vi "mark_10_config_panel.vi"(8 "Error In":errorcluster, 11 "Mark-10 Settings":T1) -> (0 "Error Out":errorcluster, 3 "Mark-10 Settings 2":T1)   [LabVIEW 2017]
uses:
  mark_10_setting_1.ctl
panel:
  in  "Cancel Button":bool
  in  "OK Button":bool
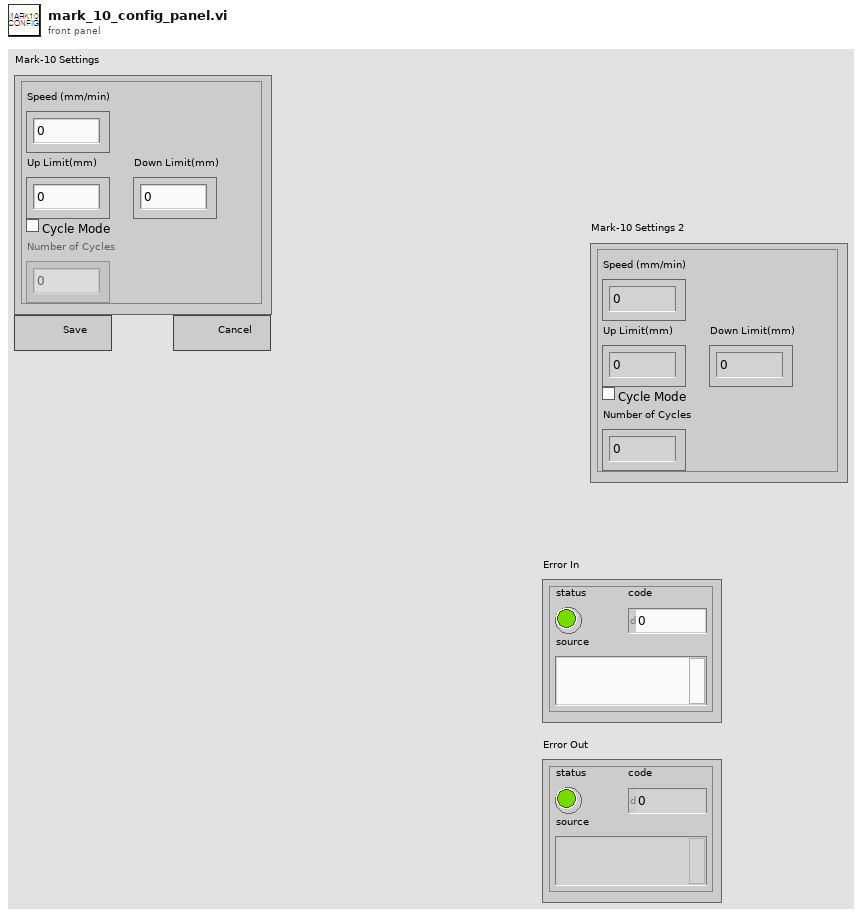
[diagram p1: front panel]
types:
  T1 = typedef "mark_10_setting_1.ctl" = cluster{"Speed (mm/min)":dbl, "Up Limit(mm)":dbl, "Down Limit(mm)":dbl, "Cycle Mode":bool, "Number of Cycles":i32, "IsConfigured":bool}
  T2 = enum8{"Enabled", "Disabled", "Disabled and Grayed Out"}
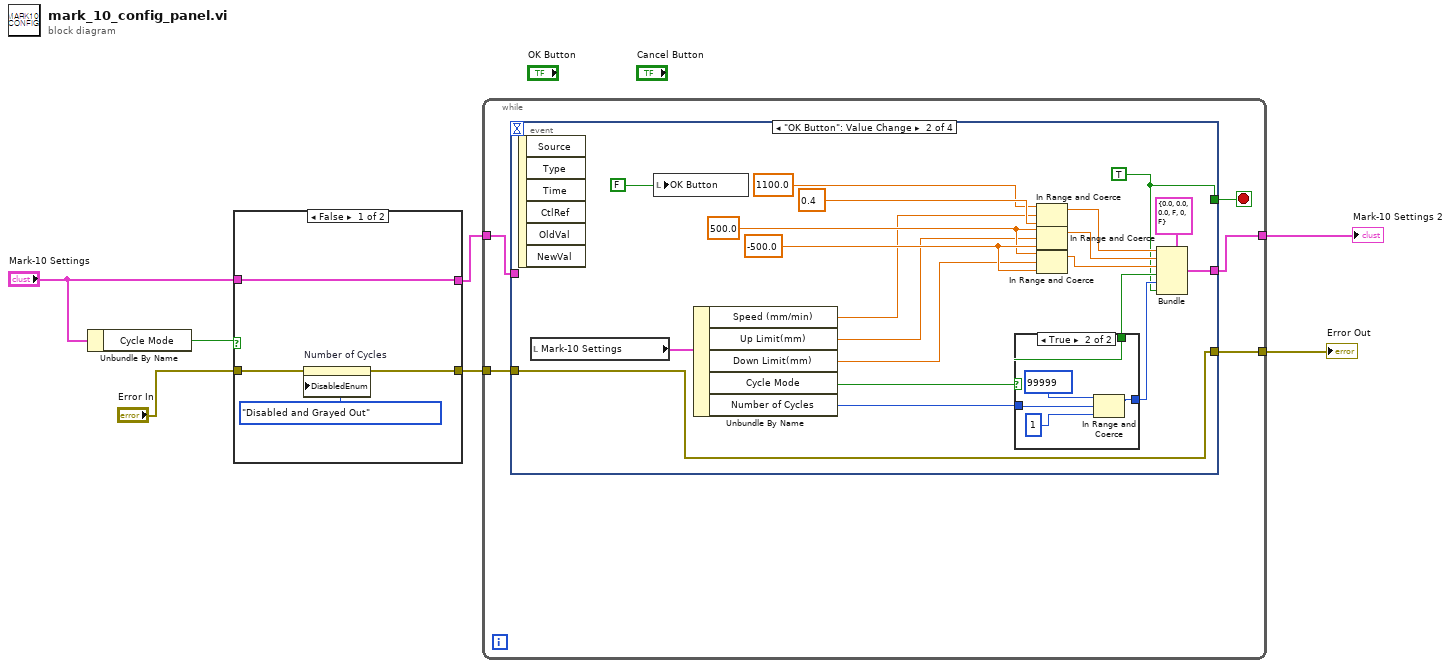
[diagram p0: block diagram]
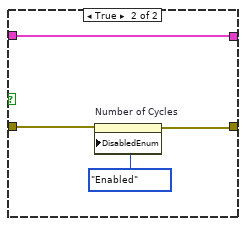
[diagram p2: hidden frame]
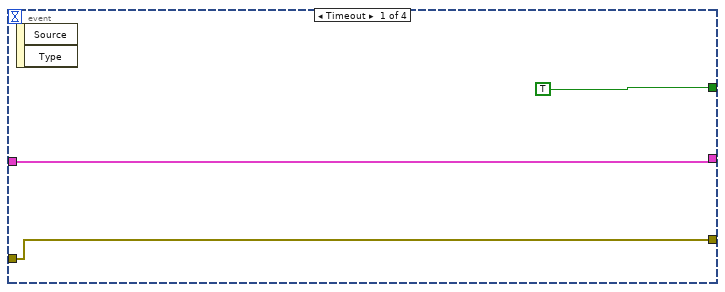
[diagram p3: hidden frame]
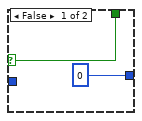
[diagram p4: hidden frame]
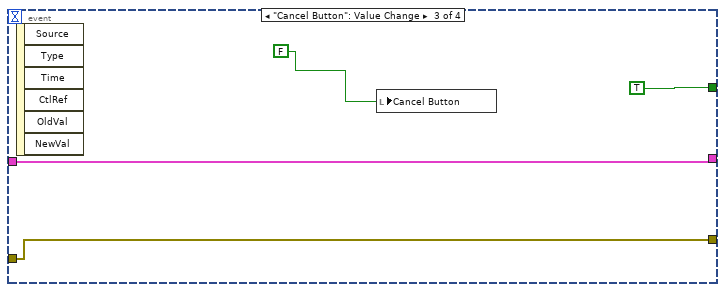
[diagram p5: hidden frame]
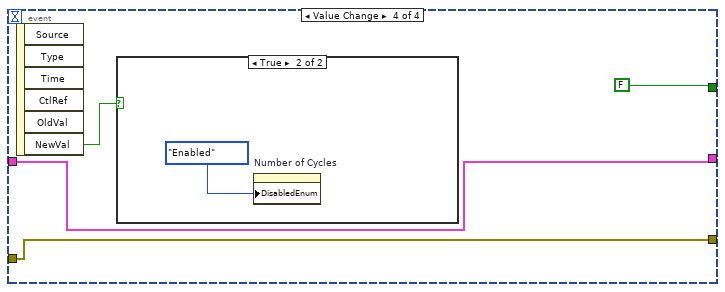
[diagram p6: hidden frame]
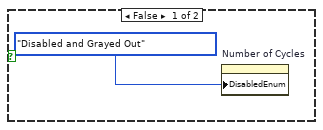
[diagram p7: hidden frame]
diagram:
  n1 = Unbundle By Name("Mark-10 Settings") -> ("Cycle Mode"=w6:bool)
  n2 = case shown="False" w6 {
    tunnel: [w10 w14] -> w4
    tunnel: "Mark-10 Settings" -> [w10 w14]
    tunnel: "Error In" -> [w9 w13]
    tunnel: [w8 w12] -> w2
    frame False {
      n3 = property on="Number of Cycles" class="DigNum (strict)"(error in=w9, "DisabledEnum"=T2."Disabled and Grayed Out" ("Disabled")) -> (error out=w8:errorcluster)  [unwired: 1 in, 1 out]
    }
    frame True {
      n4 = property on="Number of Cycles" class="DigNum (strict)"(error in=w13, "DisabledEnum"=T2."Enabled" ("Disabled")) -> (error out=w12:errorcluster)  [unwired: 1 in, 1 out]
    }
  }
  n5 = while {
    tunnel: w4 -> [w18]
    tunnel: [w20] -> w7
    tunnel: w2 -> [w17]
    tunnel: [w16] -> w1
    stop <- w19 stop-if-true
    n6 = event shown="[1] \"OK Button\": Value Change" {
      selector: _ -> [_ _ _ _]
      dyn-events: _ -> [_ _ _ _]
      timeout: _ -> [_ _ _ _]
      tunnel: [TRUE w24 TRUE FALSE] -> w19
      tunnel: [w22 w38 w52 w56] -> w20
      tunnel: w18 -> [w22 _ w52 w56]
      tunnel: w17 -> [w21 w36 w51 w55]
      tunnel: [w21 w36 w51 w55] -> w16
      event Timeout {
        n7 = event-data() -> ()  [unwired: 1 in, 2 out]
      }
      event "OK Button": Value Change {
        w42 = -500.0
        w41 = 500.0
        w24 = TRUE
        n8 = event-data() -> ()  [unwired: 1 in, 6 out]
        n9 = local read "Mark-10 Settings"() -> (w35:T1)
        n10 = local write "OK Button"(FALSE) -> ()
        n11 = Unbundle By Name(w35) -> ("Speed (mm/min)"=w30:dbl, "Up Limit(mm)"=w31:dbl, "Down Limit(mm)"=w32:dbl, "Cycle Mode"=w33:bool, "Number of Cycles"=w34:i32)
        n12 = case shown="True" w33 {
          selector: w33 -> [w44 w46]
          tunnel: [0 w50] -> w29
          tunnel: w34 -> [_ w47]
          tunnel: [w44 w46] -> w28
          frame False {
          }
          frame True {
            n13 = In Range and Coerce(upper limit=99999, x=w47, lower limit=1) -> (coerced(x)=w50:i32)  [unwired: 1 out]
          }
        }
        n14 = In Range and Coerce(upper limit=1100.0, x=w30, lower limit=0.4) -> (coerced(x)=w27:dbl)  [unwired: 1 out]
        n15 = In Range and Coerce(upper limit=w41, x=w31, lower limit=w42) -> (coerced(x)=w26:dbl)  [unwired: 1 out]
        n16 = In Range and Coerce(upper limit=w41, x=w32, lower limit=w42) -> (coerced(x)=w25:dbl)  [unwired: 1 out]
        n17 = Bundle(cluster=T1 {"Speed (mm/min)"=0.0, "Up Limit(mm)"=0.0, "Down Limit(mm)"=0.0, "Cycle Mode"=FALSE, "Number of Cycles"=0, "IsConfigured"=FALSE} ("Mark-10 Settings"), "Speed (mm/min)"=w27, "Up Limit(mm)"=w26, "Down Limit(mm)"=w25, "Cycle Mode"=w28, "Number of Cycles"=w29, "IsConfigured"=w24) -> (w38:T1)
      }
      event "Cancel Button": Value Change {
        n18 = event-data() -> ()  [unwired: 1 in, 6 out]
        n19 = local write "Cancel Button"(FALSE) -> ()
      }
      event Value Change {
        n20 = event-data() -> ("NewVal"=w57:bool)  [unwired: 1 in, 5 out]
        n21 = case shown="True" w57 {
          frame False {
            n22 = property on="Number of Cycles" class="DigNum (strict)"("DisabledEnum"=T2."Disabled and Grayed Out" ("Disabled")) -> ()  [unwired: 2 in, 2 out]
          }
          frame True {
            n23 = property on="Number of Cycles" class="DigNum (strict)"("DisabledEnum"=T2."Enabled" ("Disabled")) -> ()  [unwired: 2 in, 2 out]
          }
        }
      }
    }
  }
  "Mark-10 Settings 2" <- w7
  "Error Out" <- w1
